vi "Configure Burst.vi"(0 "RedPitaya connection in":refnum<k5>, 1 "Number of generated Signals / Burst":string, 2 "Number of repeated Bursts":string, 3 "Total time of One Burst":i32=-1, 4 "Trigger Source":u16(ring) items=["", "EXT_PE", "EXT_NE", "INT", "GATED", "IMM", "IMM BOTH"], 5 "error in":errorcluster, 6 "Channel #":u16(ring) items=["Channel 1"=1, "Channel 2"=2], 12 "timeout ms (2000)":i32=2000) -> (14 "RedPitaya connection out":refnum<k5>, 19 "error out":errorcluster)   [LabVIEW 2010, in "RedPitaya.lvlib"]
doc: "Configures the edge burst trigger mode."
uses:
  RedPitaya.lvlib
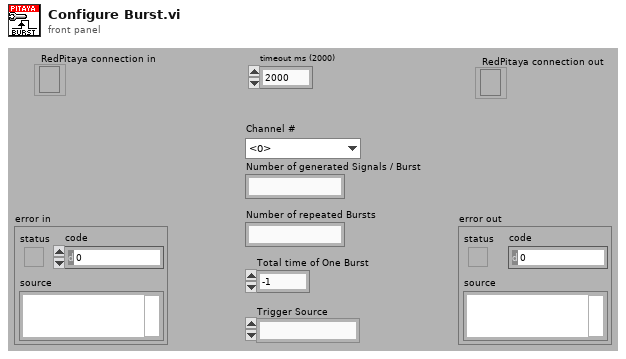
[diagram p1: front panel]
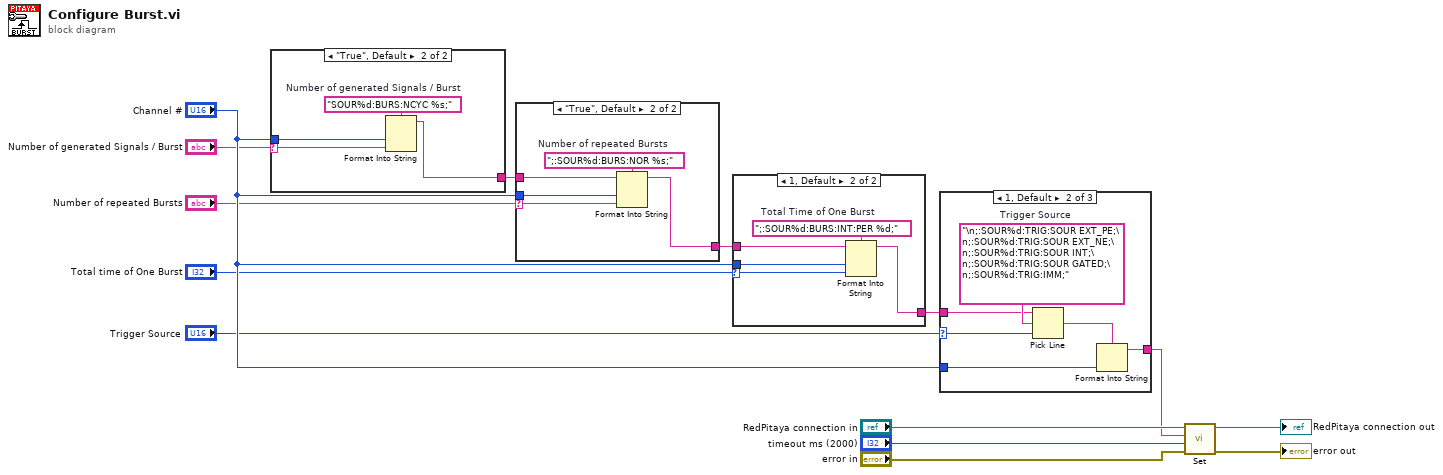
[diagram p0: block diagram]
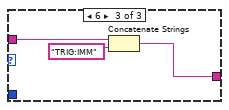
[diagram p3: hidden frame]
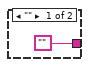
[diagram p6: hidden frame]
diagram:
  n1 = case shown="\"True\", Default" "Number of generated Signals / Burst" {
    selector: "Number of generated Signals / Burst" -> [_ w16]
    tunnel: ["" w18] -> w10
    tunnel: "Channel #" -> [_ w17]
    frame "" {
    }
    frame "True", Default {
      w19 = "SOUR%d:BURS:NCYC %s;"  # Number of generated Signals / Burst
      n2 = Format Into String(format string=w19, w17, w16) -> (resulting string=w18:string)  [unwired: 2 in, 1 out]
    }
  }
  n3 = case shown="\"True\", Default" "Number of repeated Bursts" {
    selector: "Number of repeated Bursts" -> [_ w21]
    tunnel: w10 -> [w20 w24]
    tunnel: [w20 w23] -> w9
    tunnel: "Channel #" -> [_ w22]
    frame "" {
    }
    frame "True", Default {
      w25 = ";:SOUR%d:BURS:NOR %s;"  # Number of repeated Bursts
      n4 = Format Into String(format string=w25, initial string=w24, w22, w21) -> (resulting string=w23:string)  [unwired: 1 in, 1 out]
    }
  }
  n5 = case shown="1, Default" "Total time of One Burst" {
    selector: "Total time of One Burst" -> [_ w27]
    tunnel: w9 -> [w26 w30]
    tunnel: [w26 w29] -> w8
    tunnel: "Channel #" -> [_ w28]
    frame -1 {
    }
    frame 1, Default {
      w31 = ";:SOUR%d:BURS:INT:PER %d;"  # Total Time of One Burst
      n6 = Format Into String(format string=w31, initial string=w30, w28, w27) -> (resulting string=w29:string)  [unwired: 1 in, 1 out]
    }
  }
  n7 = case shown="1, Default" "Trigger Source" {
    selector: "Trigger Source" -> [_ w34 _]
    tunnel: w8 -> [w32 w37 w41]
    tunnel: "Channel #" -> [_ w36 _]
    tunnel: [w32 w35 w39] -> w6
    frame 0 {
    }
    frame 1, Default {
      w38 = "\n;:SOUR%d:TRIG:SOUR EXT_PE;\n;:SOUR%d:TRIG:SOUR EXT_NE;\n;:SOUR%d:TRIG:SOUR INT;\n;:SOUR%d:TRIG:SOUR GATED;\n;:SOUR%d:TRIG:IMM;"  # Trigger Source
      n8 = Pick Line(string ("")=w37, multi-line string=w38, line index=w34) -> (output string=w33:string)
      n9 = Format Into String(format string=w33, w36) -> (resulting string=w35:string)  [unwired: 2 in, 1 out]
    }
    frame 6 {
      n10 = Concatenate Strings(w41, "TRIG:IMM" ("string")) -> (w39:string)
    }
  }
  n11 = call "Set.vi"("error in"="error in", "timeout ms (2000)"="timeout ms (2000)", "SCPI Message"=w6, "RedPitaya connection in"="RedPitaya connection in") -> ("error out"=→"error out":errorcluster, "RedPitaya connection out"=→"RedPitaya connection out":refnum<k5>)  [unwired: 5 in, 1 out]
